vi "DIO 10-bit.vi"(0 "DIO 0 Refnum":refnum<k21>, 1 "DIO 1 Refnum":refnum<k21>, 2 "DIO 2 Refnum":refnum<k21>, 3 "DIO 3 Refnum":refnum<k21>, 4 "DIO 4 Refnum":refnum<k21>, 5 "DIO 5 Refnum":refnum<k21>, 6 "DIO 6 Refnum":refnum<k21>, 7 "DIO 7 Refnum":refnum<k21>, 8 "DIO 8 Refnum":refnum<k21>, 9 "DIO 9 Refnum":refnum<k21>, 10 "OUT 9:0":fxp<+,10,10> format="%08b", 12 "DIR 9:0":fxp<+,10,10> format="%08b") -> (14 "IN 9:0":fxp<+,10,10> format="%08b")   [LabVIEW 2019]
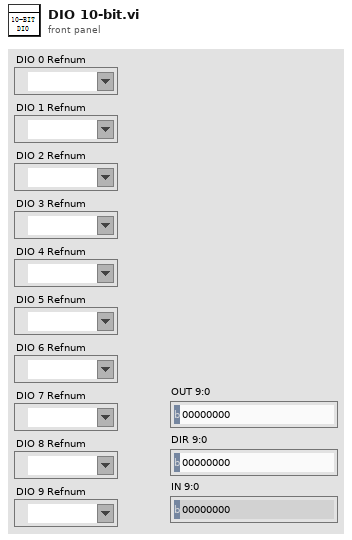
[diagram p1: front panel]
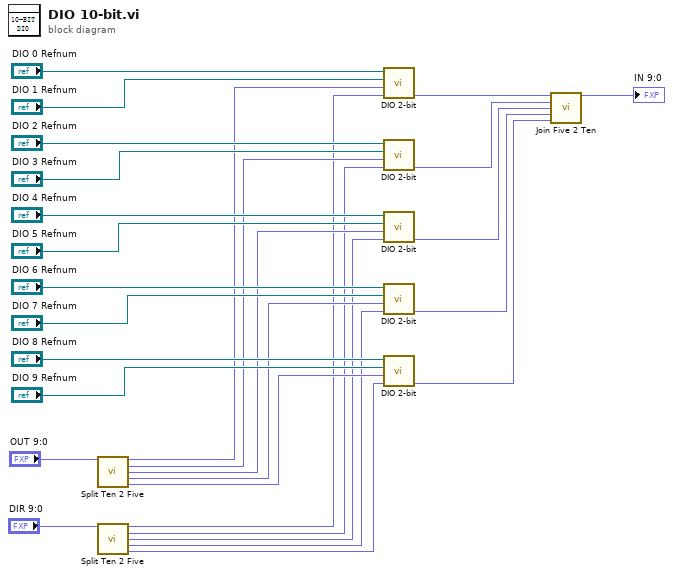
[diagram p0: block diagram]
diagram:
  n1 = call "Split Ten 2 Five.vi"("OUT 9:0"="OUT 9:0") -> ("OUT 1:0"=w17:fxp<+,2,2>, "OUT 1:0 2"=w16:fxp<+,2,2>, "OUT 1:0 3"=w15:fxp<+,2,2>, "OUT 1:0 4"=w14:fxp<+,2,2>, "OUT 1:0 5"=w13:fxp<+,2,2>)  [unwired: 10 in]
  n2 = call "Split Ten 2 Five.vi"("OUT 9:0"="DIR 9:0") -> ("OUT 1:0"=w11:fxp<+,2,2>, "OUT 1:0 2"=w10:fxp<+,2,2>, "OUT 1:0 3"=w9:fxp<+,2,2>, "OUT 1:0 4"=w8:fxp<+,2,2>, "OUT 1:0 5"=w7:fxp<+,2,2>)  [unwired: 10 in]
  n3 = call "DIO 2-bit.vi"("DIO0 Refnum"="DIO 0 Refnum", "DIO1 Refnum"="DIO 1 Refnum", "OUT 1:0"=w17, "DIR 1:0 2"=w11) -> ("IN 1:0"=w6:fxp<+,2,2>)  [unwired: 6 in]
  n4 = call "DIO 2-bit.vi"("DIO0 Refnum"="DIO 2 Refnum", "DIO1 Refnum"="DIO 3 Refnum", "OUT 1:0"=w16, "DIR 1:0 2"=w10) -> ("IN 1:0"=w5:fxp<+,2,2>)  [unwired: 6 in]
  n5 = call "DIO 2-bit.vi"("DIO0 Refnum"="DIO 4 Refnum", "DIO1 Refnum"="DIO 5 Refnum", "OUT 1:0"=w15, "DIR 1:0 2"=w9) -> ("IN 1:0"=w4:fxp<+,2,2>)  [unwired: 6 in]
  n6 = call "DIO 2-bit.vi"("DIO0 Refnum"="DIO 6 Refnum", "DIO1 Refnum"="DIO 7 Refnum", "OUT 1:0"=w14, "DIR 1:0 2"=w8) -> ("IN 1:0"=w3:fxp<+,2,2>)  [unwired: 6 in]
  n7 = call "DIO 2-bit.vi"("DIO0 Refnum"="DIO 8 Refnum", "DIO1 Refnum"="DIO 9 Refnum", "OUT 1:0"=w13, "DIR 1:0 2"=w7) -> ("IN 1:0"=w2:fxp<+,2,2>)  [unwired: 6 in]
  n8 = call "Join Five 2 Ten.vi"("OUT 1:0"=w6, "OUT 1:0 2"=w5, "OUT 1:0 3"=w4, "OUT 1:0 4"=w3, "OUT 1:0 5"=w2) -> ("OUT 9:0"=→"IN 9:0":fxp<+,10,10>)  [unwired: 10 in]
